vi "Single Trigger Type.vi"(8 "error in":errorcluster, 10 "Trigger Type":i32(ring) items=["Edge", "Pulse Width Inside", "Pulse Width Outside", "Pulse Width Less than", "Pulse Width Greater than", "Pulse Width Equal To", "Pulse Width Not Equal To", "Glitch", "Video"], 11 "Instrument Handle In":i32) -> (0 "error out":errorcluster, 3 "Instrument Handle Out":i32)   [LabVIEW 8.6, in "ZTScopeM.lvlib"]
doc: "Configure the trigger type."
uses:
  ZTScopeM.lvlib
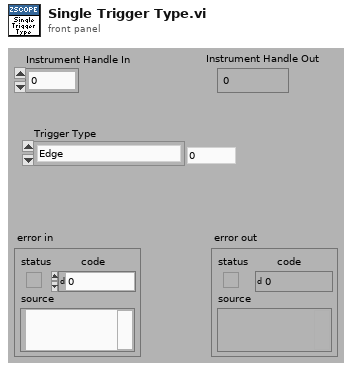
[diagram p1: front panel]
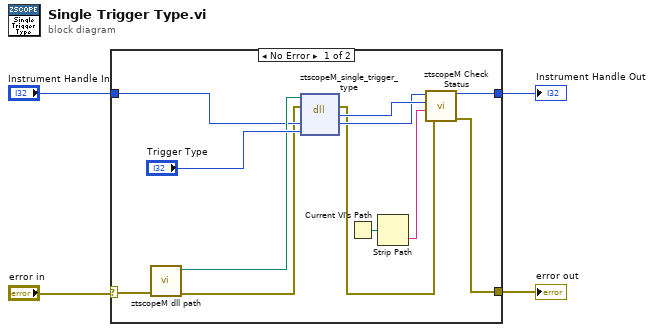
[diagram p0: block diagram]
diagram:
  n1 = case shown="No Error" "error in" {
    selector: "error in" -> [w9 w18]
    tunnel: [w11 w18] -> w3
    tunnel: [w12 w17] -> w2
    tunnel: "Instrument Handle In" -> [w7 w17]
    frame #0 {
      n2 = call "ztscopeM dll path.vi"("error in (no error)"=w9) -> ("error out"=w6:errorcluster, "<instrument>.dll path"=w8:path)  [unwired: 9 in]
      n3 = dll-call lib="C:/Projects/codedepot/Teradyne/2016-1034 Teradyne ZScope API/Software/C src/ztScopeM/ZtScopeM.dll" fn="ztscopeM_single_trigger_type" ("ztscopeM.dll:ztscopeM_single_trigger_level")(path in=w8, error in=w6, "instrumentHandle"=w7, "Trigger Type"="Trigger Type") -> (error out=w5:errorcluster, "return type"=w16:i32, "instrumentHandle"=w15:i32)  [unwired: 2 in, 1 out]
      n4 = Current VI's Path() -> (path=w14:path)
      n5 = Strip Path(path=w14) -> (name=w13:string)  [unwired: 1 out]
      n6 = call "ztscopeM Check Status.vi"("error in"=w5, "name of VI"=w13, "status (return code)"=w16, "instrument handle in"=w15) -> ("error out"=w11:errorcluster, "instrument handle out"=w12:i32)  [unwired: 2 out]
    }
    frame #1 {
    }
  }
  "Instrument Handle Out" <- w2
  "error out" <- w3
